vi "rtout_controlSignalMode.vi"(7 "Set":bool, 8 "error in":errorcluster, 9 "mode":i32, 11 "connection ID":refnum<k5>) -> (0 "error out":errorcluster, 1 "mode out":i32, 3 "connection ID":refnum<k5>)   [LabVIEW 2015, in "AMC_VIs.lvlib"]
doc: "This function retrieves or sets the real time output mode for the selected axis."
uses:
  AMC_VIs.lvlib
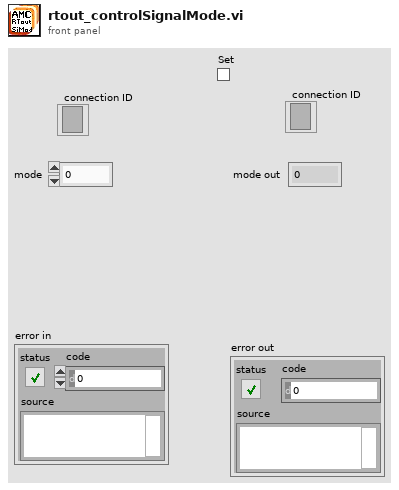
[diagram p1: front panel]
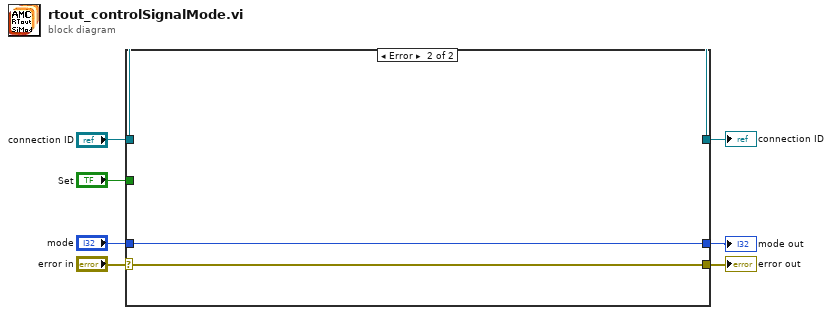
[diagram p0: block diagram]
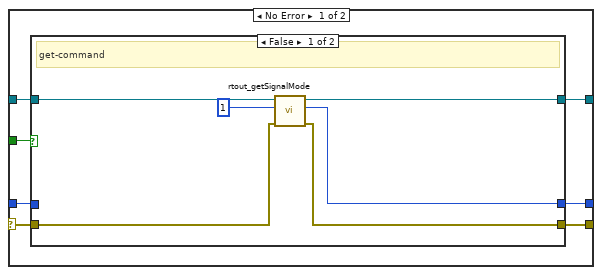
[diagram p2: hidden frame]
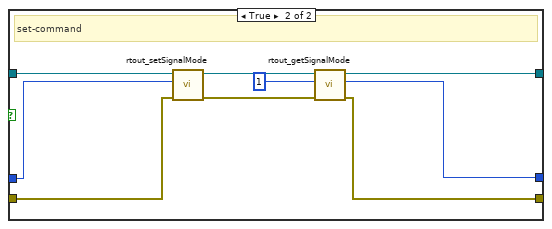
[diagram p3: hidden frame]
diagram:
  n1 = case shown="Error" "error in" {
    selector: "error in" -> [w11 w32]
    tunnel: [w9 w32] -> w7
    tunnel: "mode" -> [w13 w30]
    tunnel: [w10 w30] -> w2
    tunnel: "Set" -> [w12 _]
    tunnel: [w8 w31] -> w5
    tunnel: "connection ID" -> [w14 w31]
    frame No Error {
      n2 = case shown="False" w12 {
        tunnel: w14 -> [w20 w25]
        tunnel: w13 -> [_ w21]
        tunnel: w11 -> [w17 w29]
        tunnel: [w15 w24] -> w10
        tunnel: [w18 w27] -> w9
        tunnel: [w19 w23] -> w8
        frame False {
          # "get-command"
          n3 = call "rtout_getSignalMode.vi"("error in"=w17, "tempvalue"=1, "connection ID"=w20) -> ("error out"=w18:errorcluster, "mode"=w15:i32, "connection ID"=w19:refnum<k5>)  [unwired: 6 in]
        }
        frame True {
          # "set-command"
          n4 = call "rtout_setSignalMode.vi"("error in"=w29, "mode"=w21, "connection ID"=w25) -> ("error out"=w28:errorcluster, "connection ID"=w26:refnum<k5>)  [unwired: 7 in]
          n5 = call "rtout_getSignalMode.vi"("error in"=w28, "tempvalue"=1, "connection ID"=w26) -> ("error out"=w27:errorcluster, "mode"=w24:i32, "connection ID"=w23:refnum<k5>)  [unwired: 6 in]
        }
      }
    }
    frame Error {
    }
  }
  "error out" <- w7
  "mode out" <- w2
  "connection ID" <- w5
